vi "SOUR_POW_CORR_LEV.vi"(0 "VISA IN":refnum<visa-resource-name>, 1 "Port number":i32, 2 "Cal Power Level(dBm)":i32, 3 "Source Port":string, 5 "error in":errorcluster, 7 "Channel":i32) -> (14 "VISA Out":refnum<visa-resource-name>, 19 "error out":errorcluster)   [LabVIEW 2018, in "PNA-X.lvlib"]
doc: "SOURce<cnum>:POWer<port>:CORRection:LEVel <num>[,src] \n(Read-Write) Specifies the power level that is expected at the desired reference plane (DUT input or \noutput). This is not used for segment sweep with independent power levels or power sweeps. \nNote: Although this command still works, it is recommended that you specify cal power by setting the \ntest port power and offset value. \nParameters \n<cnum> Any existing channel number. If unspecified, value is set to 1 \n<port> Port number to correct for source power. If unspecified, value is set to 1. \n<num> Cal power level in dBm. Because this could potentially be at the output of a \ndevice-under-test, no limits are placed on this value here. It is realistically \nlimited by the specifications of the device (power sensor) that will be used for \nmeasuring the power. The power delivered to the PNA receiver must never \nexceed PNA specifications for the receiver! \n[src] String. (NOT case sensitive). Source port. Optional. Use SOUR:CAT? to \nreturn a list of valid port names. \nWhile this argument can be used to make settings for ALL ports, it is designed \nto access ports that are not simple numbers, such as \"Port 1 Src2\". Otherwise, \nthe <port> argument performs the same function. If both arguments are \nspecified, [src] takes priority. \nExamples SOUR:POW:CORR:LEV 10 \nsource1:power2:correction:level 0 dbm \nQuery Syntax SOURce:POWer:CORRection:LEVel? [src] \n1847\n\nReturn Type Numeric \nDefault 0 dBm"
uses:
  PNA-X.lvlib
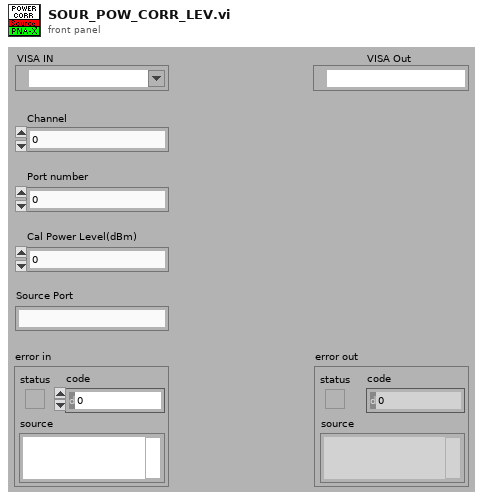
[diagram p1: front panel]
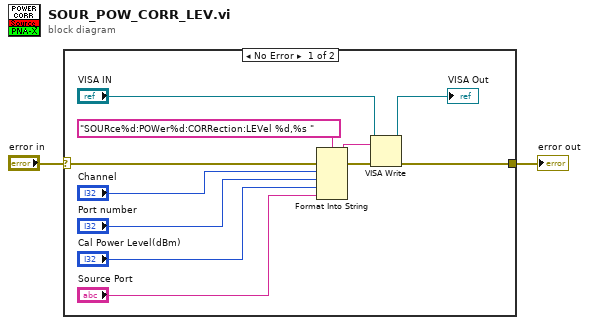
[diagram p0: block diagram]
diagram:
  n1 = case shown="No Error" "error in" {
    selector: "error in" -> [w13 w14]
    tunnel: [w8 w14] -> w1
    frame No Error {
      n2 = Format Into String(format string="SOURce%d:POWer%d:CORRection:LEVel %d,%s " ("Cmdline"), error in=w13, "Channel", "Port number", "Cal Power Level(dBm)", "Source Port") -> (resulting string=w11:string, error out=w12:errorcluster)  [unwired: 1 in]
      n3 = VISA Write(VISA resource name="VISA IN", write buffer=w11, error in (no error)=w12) -> (VISA resource name out=→"VISA Out":refnum<visa-resource-name>, error out=w8:errorcluster)  [unwired: 1 out]
    }
    frame Error {
    }
  }
  "error out" <- w1
